vi "Read commandName.vi"(8 "error in (no error)":errorcluster, 11 "CaptureSpectImage in":refnum<class "captureSpectImage.lvclass">) -> (0 "error out":errorcluster, 2 "CommandValue":T1, 3 "CaptureSpectImage out":refnum<class "captureSpectImage.lvclass">)   [LabVIEW 2016, in "Commands.lvlib" / "captureSpectImage.lvclass"]
uses:
  captureSpectImage.lvclass
  Typedefs/CommandValue.ctl
  Typedefs/EXATypedefs.lvlib
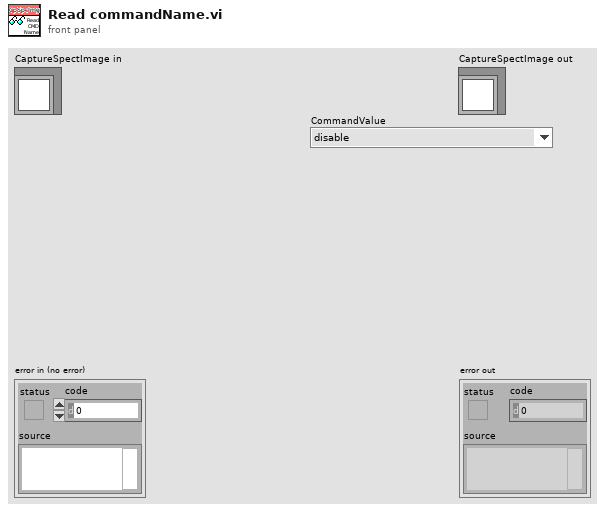
[diagram p1: front panel]
types:
  T1 = typedef "EXATypedefs.lvlib/CommandValue.ctl" = enum16{"disable", "enable", "exit", "GoToStandby", "OnHeartbeat", "OnIncomingMessagingError", "OnInterrupt", "start", "captureSpectImage", "setSpectTempSetpoint", "stopImageCapture"}
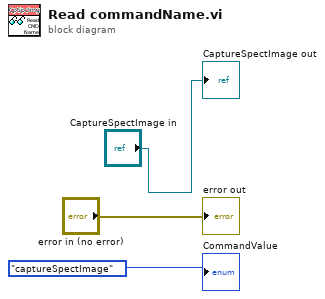
[diagram p0: block diagram]
diagram:
  "error out" <- "error in (no error)"
  "CaptureSpectImage out" <- "CaptureSpectImage in"
  "CommandValue" <- CommandValue."captureSpectImage" ("CommandValue")
